vi "Open Parent Class.vi"(8 "error in (no error)":errorcluster, 11 "QControl Creation in":refnum<class "QControl Creation.lvclass">) -> (0 "error out":errorcluster, 3 "QControl Creation out":refnum<class "QControl Creation.lvclass">)   [LabVIEW 2023, in "QControl Creation.lvclass"]
doc: "<b> </b> <b> </b>\n©2016 Q Software Innovations, LLC (QSI)\nwritten by Quentin Alldredge\nproduced in LabVIEW 2015\n\nsupport@qsoftwareinnovations.com\nwww.qsoftwareinnovations.com\n\nAll rights reserved.\n\nRedistribution and use in source and binary forms, with or without modification, are permitted provided that the following conditions are met:\n\n * Redistributions of source code must retain the above copyright notice, this list of conditions and the following disclaimer.\n * Redistributions in binary form must reproduce the above copyright notice, this list of conditions and the following disclaimer in the documentation and/or other materials provided with the distribution.\n * Neither the name of Q Software Innovations, LLC. nor the names of its contributors may be used to endorse or promote products derived from this software without specific prior written permission.\n\nTHIS SOFTWARE IS PROVIDED BY THE COPYRIGHT HOLDERS AND CONTRIBUTORS \"AS IS\" AND ANY EXPRESS OR IMPLIED WARRANTIES, INCLUDING, BUT NOT LIMITED TO, THE IMPLIED WARRANTIES OF MERCHANTABILITY AND FITNESS FOR A PARTICULAR PURPOSE ARE DISCLAIMED. IN NO EVENT SHALL THE COPYRIGHT OWNER OR CONTRIBUTORS BE LIABLE FOR ANY DIRECT, INDIRECT, INCIDENTAL, SPECIAL, EXEMPLARY, OR CONSEQUENTIAL DAMAGES (INCLUDING, BUT NOT LIMITED TO, PROCUREMENT OF SUBSTITUTE GOODS OR SERVICES; LOSS OF USE, DATA, OR PROFITS; OR BUSINESS INTERRUPTION) HOWEVER CAUSED AND ON ANY THEORY OF LIABILITY, WHETHER IN CONTRACT, STRICT LIABILITY, OR TORT (INCLUDING NEGLIGENCE OR OTHERWISE) ARISING IN ANY WAY OUT OF THE USE OF THIS SOFTWARE, EVEN IF ADVISED OF THE POSSIBILITY OF SUCH DAMAGE."
uses:
  QControl Creation.lvclass
  QControl Creation.lvclass/QControl Creation.ctl
  New QControl Info/New QControl Info.lvclass/New QControl Info.ctl
  New QControl Info/Read App Refnum.vi
  New QControl Info/Read Parent Class Path.vi
  New QControl Info/New QControl Info.lvclass
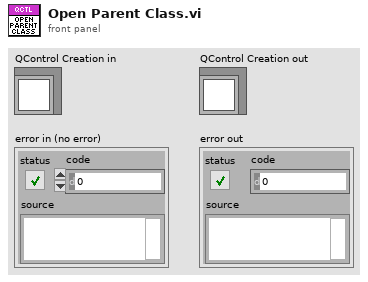
[diagram p1: front panel]
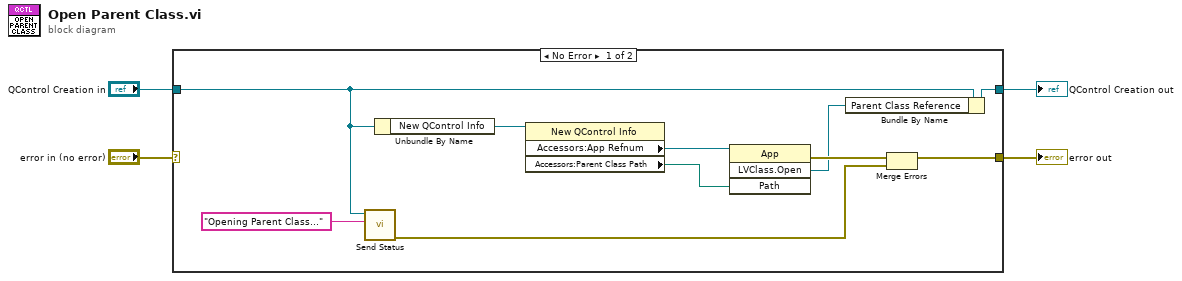
[diagram p0: block diagram]
diagram:
  n1 = case shown="No Error" "error in (no error)" {
    selector: "error in (no error)" -> [_ w15]
    tunnel: "QControl Creation in" -> [w11 w16]
    tunnel: [w9 w15] -> w3
    tunnel: [w13 w16] -> w2
    frame No Error {
      n2 = call "Send Status.vi"("Status"="Opening Parent Class...", "QControl Creation in"=w11) -> ("error out (dup)"=w8:errorcluster)  [unwired: 8 in, 1 out]
      n3 = Unbundle By Name(w11) -> ("New QControl Info"=w7:refnum<data-value>)
      n4 = property class="New QControl Info"(reference=w7) -> ("Accessors:App Refnum"=w5:refnum<vi>, "Accessors:Parent Class Path"=w6:path)  [unwired: 1 in, 2 out]
      n5 = invoke class="App" method="LVClass.Open"(reference=w5, "Path"=w6) -> (error out=w14:errorcluster, "LVClass.Open"=w12:refnum<vi>)  [unwired: 2 in, 2 out]
      n6 = Bundle By Name(cluster=w11, "Parent Class Reference"=w12) -> (w13:refnum<class "QControl Creation.lvclass">)
      n7 = Merge Errors(w14, w8) -> (w9:errorcluster)
    }
    frame Error {
    }
  }
  "error out" <- w3
  "QControl Creation out" <- w2
